vi "SortHawkeyeList.vi"(8 "error in (no error)":errorcluster, 11 "Hawkeye File Path":path=path "C:/sw-deps-monitor/Source") -> (0 "error out":errorcluster, 3 "Hawkeye File Path Out":path)   [LabVIEW 2019, in "DepsWatch.lvlib"]
uses:
  DepsWatch.lvlib
  <vilib>/Utility/config.llb/Write Key (String).vi
  <vilib>/Utility/config.llb/NI_LVConfig.lvlib
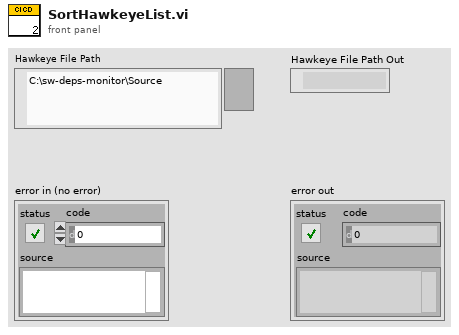
[diagram p1: front panel]
types:
  T1 = typedef "NI_LVConfig.lvlib/Config Data RefNum.ctl" = refnum<k1>
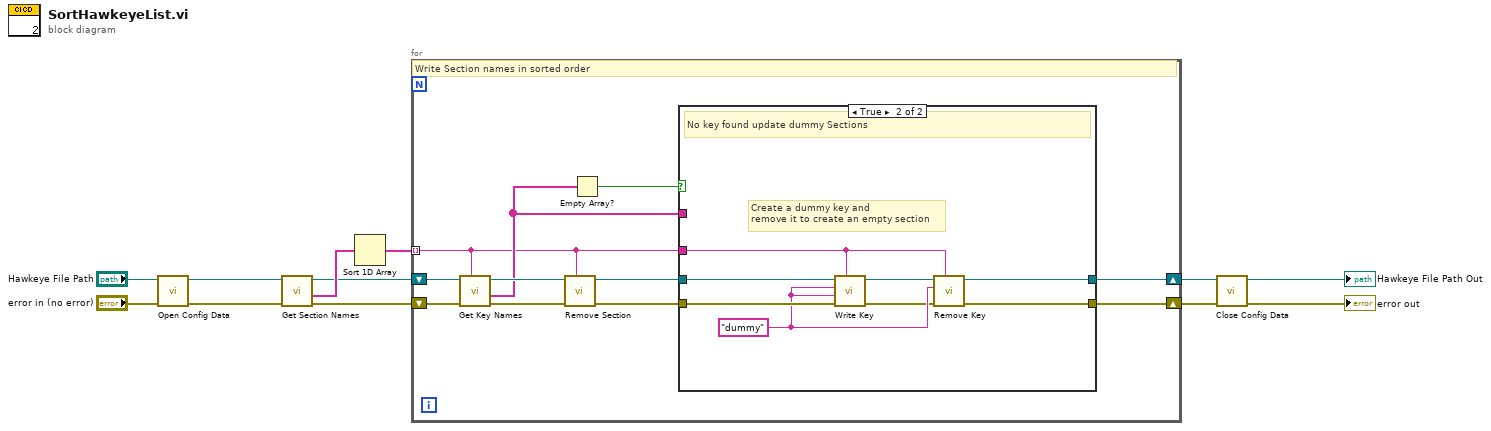
[diagram p0: block diagram]
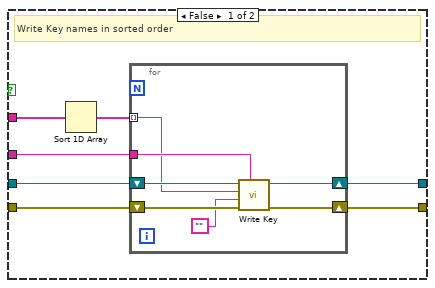
[diagram p2: hidden frame]
diagram:
  n1 = call <vilib>:"Open Config Data.vi"("error in (no error)"="error in (no error)", "configuration file path"="Hawkeye File Path") -> ("error out"=w9:errorcluster, "refnum"=w10:T1)  [unwired: 7 in, 1 out]
  n2 = call <vilib>:"Get Section Names.vi"("error in (no error)"=w9, "refnum"=w10) -> ("error out"=w7:errorcluster, "section names"=w8:string[], "refnum out"=w6:T1)  [unwired: 7 in]
  n3 = Sort 1D Array(array=w8) -> (sorted array=w2:string[])
  n4 = for {
    tunnel: w2 -> [w14] mode=indexing
    shift-right: [w16] -> w4
    shift-left: w7 -> [w23]
    shift-right: [w17] -> w5
    shift-left: w6 -> [w20]
    # "Write Section names in sorted order"
    n5 = call <vilib>:"Get Key Names.vi"("section"=w14, "error in (no error)"=w23, "refnum"=w20) -> ("error out"=w22:errorcluster, "key names"=w15:string[], "refnum out"=w21:T1)  [unwired: 5 in, 1 out]
    n6 = call <vilib>:"Remove Section.vi"("section"=w14, "error in (no error)"=w22, "refnum"=w21) -> ("error out"=w18:errorcluster, "refnum out"=w19:T1)  [unwired: 6 in, 1 out]
    n7 = Empty Array?(array=w15) -> (empty?=w13:bool)
    n8 = case shown="True" w13 {
      tunnel: w19 -> [w30 w45]
      tunnel: w18 -> [w29 w44]
      tunnel: [w28 w41] -> w17
      tunnel: [w27 w42] -> w16
      tunnel: w15 -> [w26 _]
      tunnel: w14 -> [w25 w38]
      frame False {
        # "Write Key names in sorted order"
        n9 = Sort 1D Array(array=w26) -> (sorted array=w24:string[])
        n10 = for {
          tunnel: w24 -> [w32] mode=indexing
          shift-right: [w35] -> w28
          shift-left: w30 -> [w37]
          shift-right: [w34] -> w27
          shift-left: w29 -> [w36]
          tunnel: w25 -> [w33]
          n11 = call-poly <vilib>:"Write Key.vi"("section"=w33, "error in (no error)"=w36, "value"="", "key"=w32, "refnum"=w37) -> ("error out"=w34:errorcluster, "refnum out"=w35:T1)  [unwired: 4 in, 1 out]
        }
      }
      frame True {
        w43 = "dummy" ("key")
        # "Create a dummy key and\nremove it to create an empty section"
        # "No key found update dummy Sections"
        n12 = call-poly <vilib>:"Write Key.vi"("section"=w38, "error in (no error)"=w44, "value"=w43, "key"=w43, "refnum"=w45) -> ("error out"=w40:errorcluster, "refnum out"=w39:T1)  [unwired: 4 in, 1 out]
        n13 = call <vilib>:"Remove Key.vi"("section"=w38, "error in (no error)"=w40, "key"=w43, "refnum"=w39) -> ("error out"=w42:errorcluster, "refnum out"=w41:T1)  [unwired: 5 in, 1 out]
      }
    }
  }
  n14 = call <vilib>:"Close Config Data.vi"("error in (no error)"=w4, "refnum"=w5) -> ("error out"=→"error out":errorcluster, "file path"=→"Hawkeye File Path Out":path)  [unwired: 8 in]
